vi "Get Result by Position.vi"(8 "error in (no error)":errorcluster, 10 "Position":i32, 11 "Application in":refnum<class "Application.lvclass">) -> (0 "error out":errorcluster, 2 "Test Results":T1={"Position"=0, "Pass"=TRUE, "Fail Codes"=""})   [LabVIEW 2017, in "Application.lvlib" / "Application.lvclass"]
doc: "Returns the current result for an existing position."
uses:
  Application.lvclass
  Properties/Test Result -- Cluster.ctl
  Properties/App Properties.lvclass
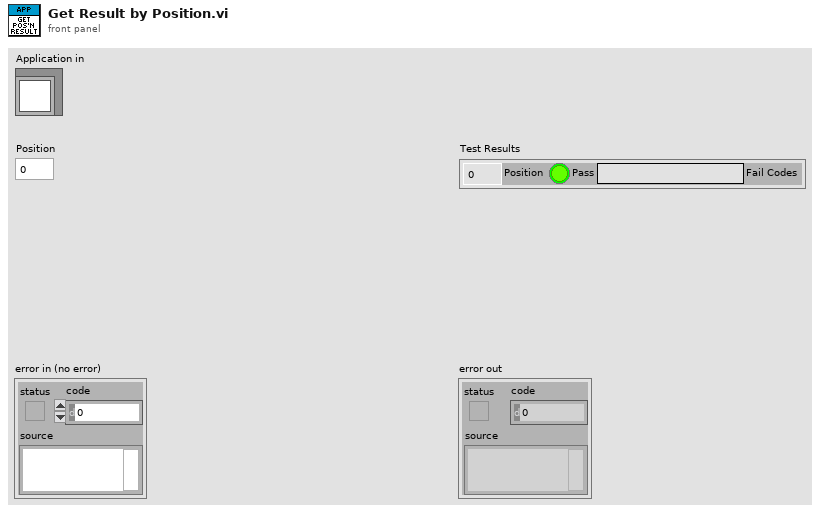
[diagram p1: front panel]
types:
  T1 = typedef "Application.lvlib/App Properties.lvclass/Test Result -- Cluster.ctl" = cluster{"Position":i32, "Pass":bool, "Fail Codes":string}
  T2 = typedef "Application.lvlib/App Properties.lvclass/Class Properties -- Cluster.ctl" = cluster{"UUT Info":T3[], "Test Information":refnum<vi>, "Gold Board":refnum<class "Golden Board.lvclass">, "Test Recipe":refnum<class "Test Recipe.lvclass">, "Instruments":refnum<class "Instrument.lvclass">[], "Mode":T4, "Test Results":T1[], "Station Config":refnum<class "Station Config.lvclass">, "Variable Engine":refnum<class "Variable Engine.lvclass">}
  T3 = typedef "Application.lvlib/App Properties.lvclass/UUT Reference -- Cluster.ctl" = cluster{"Serial Number Reference":refnum<vi>, "Status Message Reference":refnum<vi>}
  T4 = typedef "Application.lvlib/Application.lvclass/Op Mode -- Enum.ctl" = u16
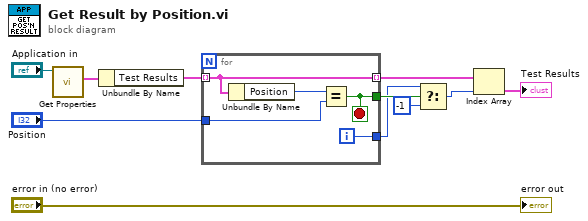
[diagram p0: block diagram]
diagram:
  n1 = call "Get Properties.vi"("Acrobat Template in"="Application in") -> ("Class Properties"=w10:T2)  [unwired: 8 in, 2 out]
  n2 = Unbundle By Name(w10) -> ("Test Results"=w8:T1[])
  n3 = for {
    tunnel: w8 -> [w16] mode=indexing
    tunnel: [w16] -> w4 mode=indexing
    tunnel: "Position" -> [w14]
    tunnel: [w13] -> w2
    tunnel: [w12] -> w3
    i -> [w13]
    stop <- w12 stop-if-true
    n4 = Unbundle By Name(w16) -> ("Position"=w15:i32)
    n5 = Equal?(x=w15, y=w14) -> (x = y?=w12:bool)
  }
  n6 = Select(t=w2, s=w3, f=-1) -> (s? t:f=w6:i32)
  n7 = Index Array(array=w4, index=w6) -> (element=→"Test Results":T1)
  "error out" <- "error in (no error)"
